vi "Ignore Files.vi"(8 "Error In":errorcluster, 9 "All Files":path[](array[path]), 10 "All Folders":path[](array[path]), 11 "Configuration":T1) -> (0 "Error Out":errorcluster, 1 "All Files":path[](array[path]), 2 "All Folders":path[](array[path]), 3 "Configuration":T1)   [LabVIEW 2011, in "LVH-Build-Tools.lvlib"]
uses:
  LVH-Build-Tools.lvlib
  Type Defs/Configuration.ctl
  Type Defs/Install Configuration.ctl
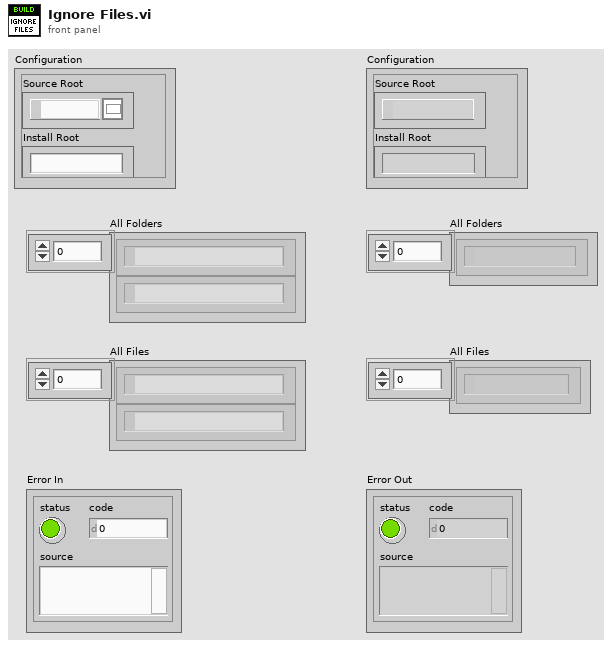
[diagram p1: front panel]
types:
  T1 = typedef "LVH-Build-Tools.lvlib/Configuration.ctl" = cluster{"Source Root":path, "Install Root":string, "Components":string[], "Ignore":string[], "Config Files":path[], "LV Directories":path[], "Install Paths":T2}
  T2 = typedef "LVH-Build-Tools.lvlib/Install Configuration.ctl" = cluster{"LabVIEW Directory":path, "Project Source Config":path}
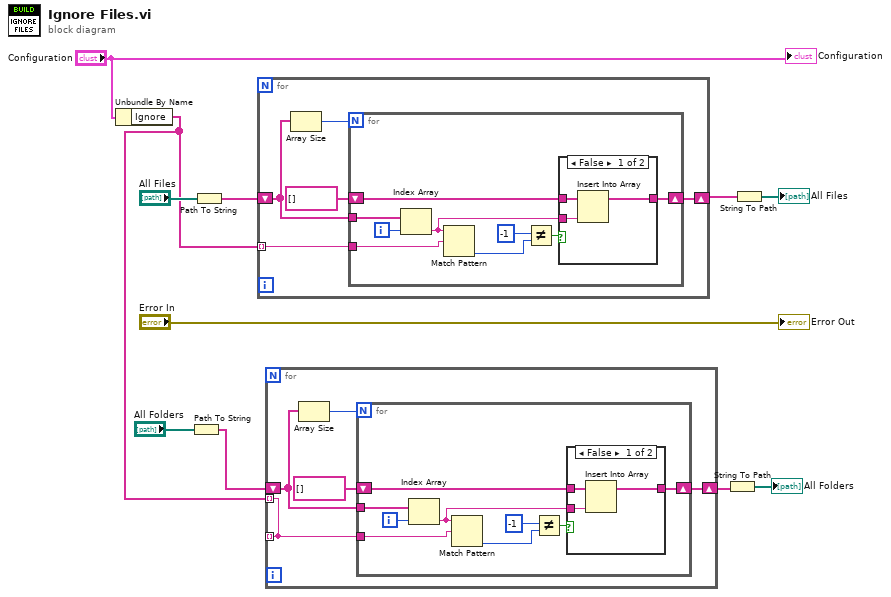
[diagram p0: block diagram]
diagram:
  n1 = Unbundle By Name("Configuration") -> ("Ignore"=w2:string[])
  n2 = Path To String(path="All Folders") -> (string=w5:string[])
  n3 = Path To String(path="All Files") -> (string=w10:string[])
  n4 = for {
    tunnel: w2 -> [w16] mode=indexing
    shift-right: [w12] -> w9
    shift-left: w10 -> [w15]
    n5 = Array Size(array=w15) -> (size(s)=w14:i32)
    n6 = for {
      N: w14 -> [_]
      tunnel: w15 -> [w24]
      tunnel: w16 -> [w25]
      shift-right: [w20] -> w12
      shift-left: string[] [] -> [w22]
      i -> [w23]
      n7 = Index Array(array=w24, index=w23) -> (element=w21:string)
      n8 = Match Pattern(string=w21, regular expression=w25) -> (offset past match=w17:i32)  [unwired: 1 in, 3 out]
      n9 = Not Equal?(x=-1 ("y"), y=w17) -> (x != y?=w19:bool)
      n10 = case shown="False" w19 {
        tunnel: w22 -> [w28 w29]
        tunnel: w21 -> [w27 _]
        tunnel: [w26 w29] -> w20
        frame False {
          n11 = Insert Into Array(array=w28, new element=w27) -> (w26:string[])  [unwired: 1 in]
        }
        frame True {
          # "Ignore File"
        }
      }
    }
  }
  n12 = for {
    tunnel: [w30] -> _ mode=indexing
    shift-right: [w31] -> w4
    shift-left: w5 -> [w34]
    tunnel: w2 -> [w30] mode=indexing
    n13 = Array Size(array=w34) -> (size(s)=w33:i32)
    n14 = for {
      N: w33 -> [_]
      tunnel: w34 -> [w42]
      tunnel: w30 -> [w43]
      shift-right: [w38] -> w31
      shift-left: string[] [] -> [w40]
      i -> [w41]
      n15 = Index Array(array=w42, index=w41) -> (element=w39:string)
      n16 = Match Pattern(string=w39, regular expression=w43) -> (offset past match=w35:i32)  [unwired: 1 in, 3 out]
      n17 = Not Equal?(x=-1 ("y"), y=w35) -> (x != y?=w37:bool)
      n18 = case shown="False" w37 {
        tunnel: w40 -> [w46 w47]
        tunnel: w39 -> [w45 _]
        tunnel: [w44 w47] -> w38
        frame False {
          n19 = Insert Into Array(array=w46, new element=w45) -> (w44:string[])  [unwired: 1 in]
        }
        frame True {
          # "Ignore File"
        }
      }
    }
  }
  n20 = String To Path(string=w4) -> (path=→"All Folders":path[])
  n21 = String To Path(string=w9) -> (path=→"All Files":path[])
  "Error Out" <- "Error In"
  "Configuration" <- "Configuration"
